vi "Write Method.vi"(10 "Method":T1, 11 "Switching Time in":refnum<class "Switching Time.lvclass">) -> (3 "Switching Time out":refnum<class "Switching Time.lvclass">)   [LabVIEW 2020, in "Switching Time.lvclass"]
uses:
  Switching Time.lvclass
  Controls/Method.ctl
  Switching Time.lvclass/Switching Time.ctl
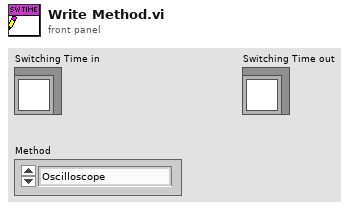
[diagram p1: front panel]
types:
  T1 = typedef "Switching Time.lvclass/Method.ctl" = enum16{"Oscilloscope", "Spectrum Analyzer"}
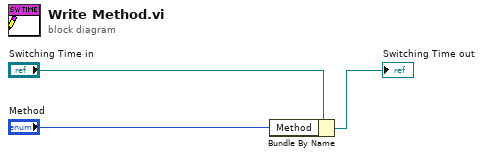
[diagram p0: block diagram]
diagram:
  n1 = Bundle By Name(cluster="Switching Time in", "Method"="Method") -> (→"Switching Time out":refnum<class "Switching Time.lvclass">)
